vi "Merge_single_configuration.vi"(9 "UseAMO":bool, 10 "Conf.set":u8, 11 "Unit selection":u8) -> (3 "Array":u8[][](array[numeric]))   [LabVIEW 2013]
panel:
  # "make inputs obligaroty!\nso you see all the instances as errors\nif adding more configs"
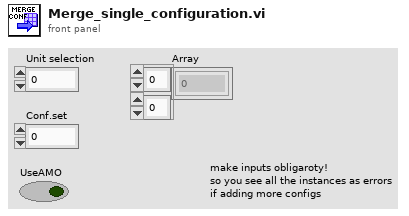
[diagram p1: front panel]
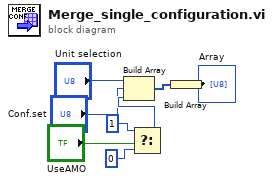
[diagram p0: block diagram]
diagram:
  n1 = Select(t=u8 1 ("Configuration set"), s="UseAMO", f=u8 0 ("Configuration set")) -> (s? t:f=w8:u8)
  n2 = Build Array("Unit selection", "Conf.set", w8) -> (w3:u8[])
  n3 = Build Array(w3) -> (→"Array":u8[][])
